vi "SelectCamera.vi"(8 "error in (no error)":errorcluster, 11 "CameraControlViewer in":refnum<class "CameraControlViewer.lvclass">) -> (0 "error out":errorcluster, 2 "CameraSettingsPath":path, 3 "CameraControlViewer out":refnum<class "CameraControlViewer.lvclass">)   [LabVIEW 2011, in "Views.lvlib" / "Camera.lvlib" / "CameraControlViewer.lvclass"]
uses:
  CameraControlViewer.lvclass
  CameraControlViewer.lvclass/CameraControlViewer.ctl
  Tools/Filing/FileSystem/FileSystem.lvclass
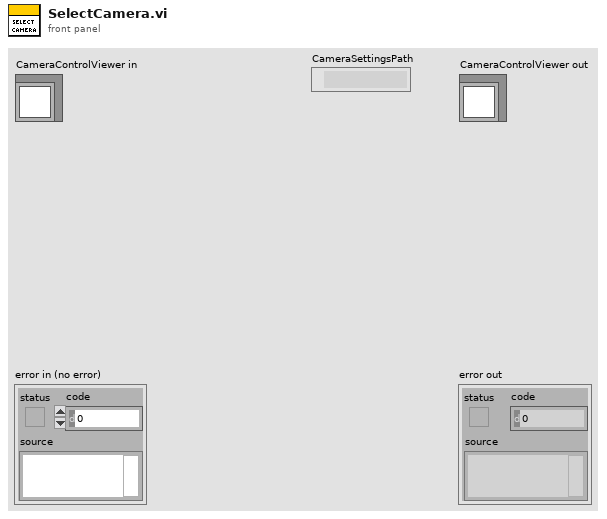
[diagram p1: front panel]
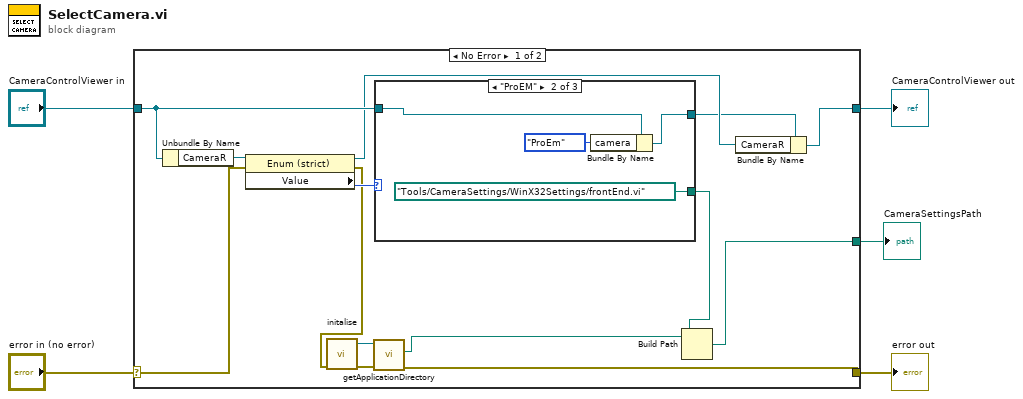
[diagram p0: block diagram]
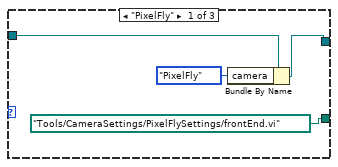
[diagram p2: hidden frame]
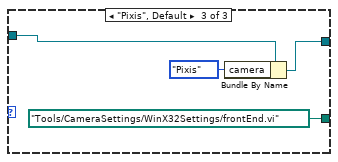
[diagram p3: hidden frame]
diagram:
  n1 = case shown="No Error" "error in (no error)" {
    selector: "error in (no error)" -> [w18 w33]
    tunnel: [w8 w33] -> w4
    tunnel: [w6 w32] -> w2
    tunnel: "CameraControlViewer in" -> [w11 w32]
    tunnel: [w12 _] -> w1
    frame No Error {
      n2 = Unbundle By Name(w11) -> ("CameraR"=w19:refnum<vi>)
      n3 = property class="Enum (strict)"(reference=w19, error in=w18) -> (reference out=w10:refnum<vi>, error out=w9:errorcluster, "Value"=w17:enum16{"Pixis", "ProEM", "PixelFly"})
      n4 = call "initalise.vi"("error in (no error)"=w9) -> ("error out"=w15:errorcluster, "FileSystem out"=w16:refnum<class "FileSystem.lvclass">)  [unwired: 9 in]
      n5 = call-dynamic "getApplicationDirectory.vi"("error in (no error)"=w15, "FileSystem.lvclass in"=w16) -> ("error out"=w8:errorcluster, "ApplicationDirectory"=w14:path)  [unwired: 7 in, 1 out]
      n6 = case shown="\"ProEM\"" w17 {
        tunnel: [path "Tools/CameraSettings/PixelFlySettings/frontEnd.vi" path "Tools/CameraSettings/WinX32Settings/frontEnd.vi" path "Tools/CameraSettings/WinX32Settings/frontEnd.vi"] -> w13
        tunnel: [w21 w24 w28] -> w7
        tunnel: w11 -> [w22 w25 w29]
        frame "PixelFly" {
          n7 = Bundle By Name(cluster=w22, "camera"=enum16{"PixelFly", "ProEm", "Pixis"}."PixelFly") -> (w21:refnum<class "CameraControlViewer.lvclass">)
        }
        frame "ProEM" {
          n8 = Bundle By Name(cluster=w25, "camera"=enum16{"PixelFly", "ProEm", "Pixis"}."ProEm") -> (w24:refnum<class "CameraControlViewer.lvclass">)
        }
        frame "Pixis", Default {
          n9 = Bundle By Name(cluster=w29, "camera"=enum16{"PixelFly", "ProEm", "Pixis"}."Pixis") -> (w28:refnum<class "CameraControlViewer.lvclass">)
        }
      }
      n10 = Build Path(base path=w14, name or relative path=w13) -> (appended path=w12:path)
      n11 = Bundle By Name(cluster=w7, "CameraR"=w10) -> (w6:refnum<class "CameraControlViewer.lvclass">)
    }
    frame Error {
    }
  }
  "error out" <- w4
  "CameraControlViewer out" <- w2
  "CameraSettingsPath" <- w1
